vi "get DC test parameters.vi"(8 "error in (no error)":errorcluster, 10 "Step":T2=1 min=1 max=99 step=1, 11 "VISA Refnum in":refnum<visa-resource-name>) -> (0 "error out":errorcluster, 3 "VISA Refnum out":refnum<visa-resource-name>, 5 "DC Parameters":T1 {"Voltage Level [V]" min=50 max=6000 step=1 format="%.3p"; "Hi Limit [A]" min=1e-07 max=0.01 step=1e-07 format="%.2p"; "Test Time [s]" min=0.0 max=999.0 step=0.1 format="%.1p"; "Dwell Time [s]" min=0.0 max=999.0 step=0.1 format="%.1p"; "Lo Limit [A]" min=0.0 max=0.01 step=1e-06 format="%.2p"; "ARC Limit [A]" min=0.0 max=0.01 step=0.001 format="%.1p"; "Ramp Time [s]" min=0.0 max=999.0 step=0.1 format="%.1p"; "Fall Time [s]" min=0.0 max=999.0 step=0.1 format="%.1p"})   [LabVIEW 2025]
uses:
  <instrlib>/Chroma 19052/Public/Utility/Type Def/steps--numeric.ctl
  DC parameters--cluster.ctl
  <instrlib>/Chroma 19052/Public/Utility/Type Def/AC-DC-IR modes--ring.ctl
  <instrlib>/Chroma 19052/Public/Utility/Type Def/AC-DC modes--ring.ctl
  <instrlib>/Chroma 19052/Public/Utility/Type Def/DC-IR modes--ring.ctl
  <instrlib>/Chroma 19052/Chroma 19052.lvlib
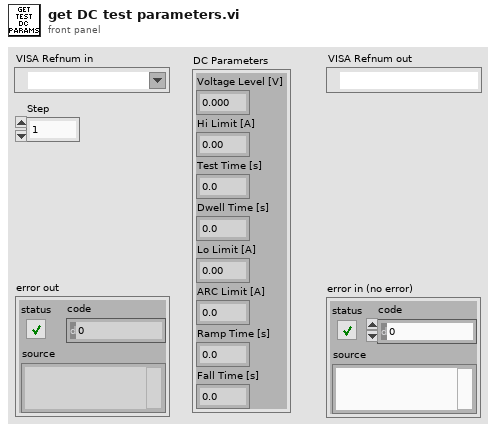
[diagram p1: front panel]
types:
  T1 = typedef "DC parameters--cluster.ctl" = cluster{"Voltage Level [V]":u16, "Hi Limit [A]":dbl, "Test Time [s] ":dbl, "Dwell Time [s]":dbl, "Lo Limit [A]":dbl, "ARC Limit [A]":dbl, "Ramp Time [s] ":dbl, "Fall Time [s]":dbl}
  T2 = typedef "Chroma 19052.lvlib/steps--numeric.ctl" = u8
  T3 = typedef "DC-IR modes--ring.ctl" = u16
  T4 = typedef "AC-DC modes--ring.ctl" = i32
  T5 = typedef "AC-DC-IR modes--ring.ctl" = u16
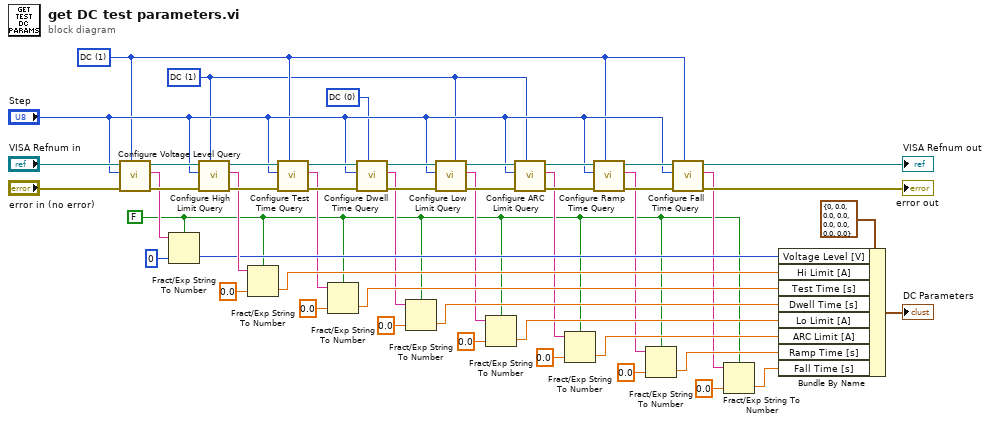
[diagram p0: block diagram]
diagram:
  w1 = FALSE
  w30 = T3 0 items=["DC", "IR"] ("Mode")
  w28 = T4 1 items=["AC", "DC"] ("Mode")
  w29 = T5 1 items=["AC", "DC", "IR"] ("Mode")
  n1 = call <instrlib>:"Configure Voltage Level Query.vi"("Mode"=w29, "error in (no error)"="error in (no error)", "Step"="Step", "VISA resource name"="VISA Refnum in") -> ("error out"=w38:errorcluster, "Voltage value [V]"=w25:string, "VISA resource name out"=w35:refnum<visa-resource-name>)  [unwired: 5 in]
  n2 = Fract/Exp String To Number(use system decimal point (T)=w1, string=w25, default (0 dbl)=u16 0 ("Voltage Level [V]")) -> (number=w21:u16)  [unwired: 1 in, 1 out]
  n3 = call <instrlib>:"Configure High Limit Query.vi"("Mode"=w28, "error in (no error)"=w38, "Step"="Step", "VISA resource name"=w35) -> ("error out"=w45:errorcluster, "High value [A]"=w22:string, "VISA resource name out"=w46:refnum<visa-resource-name>)  [unwired: 5 in]
  n4 = Fract/Exp String To Number(use system decimal point (T)=w1, string=w22, default (0 dbl)=0.0 ("Voltage Level [V]")) -> (number=w20:dbl)  [unwired: 1 in, 1 out]
  n5 = call <instrlib>:"Configure Test Time Query.vi"("Mode"=w29, "error in (no error)"=w45, "Step"="Step", "VISA resource name"=w46) -> ("error out"=w48:errorcluster, "Test Time value [s]"=w13:string, "VISA resource name out"=w32:refnum<visa-resource-name>)  [unwired: 5 in]
  n6 = Fract/Exp String To Number(use system decimal point (T)=w1, string=w13, default (0 dbl)=0.0 ("Voltage Level [V]")) -> (number=w12:dbl)  [unwired: 1 in, 1 out]
  n7 = call <instrlib>:"Configure Dwell Time Query.vi"("Mode"=w30, "error in (no error)"=w48, "Step"="Step", "VISA resource name"=w32) -> ("error out"=w47:errorcluster, "Dwell time value [s]"=w11:string, "VISA resource name out"=w49:refnum<visa-resource-name>)  [unwired: 5 in]
  n8 = Fract/Exp String To Number(use system decimal point (T)=w1, string=w11, default (0 dbl)=0.0 ("Voltage Level [V]")) -> (number=w10:dbl)  [unwired: 1 in, 1 out]
  n9 = call <instrlib>:"Configure Low Limit Query.vi"("Mode"=w28, "error in (no error)"=w47, "Step"="Step", "VISA resource name"=w49) -> ("error out"=w39:errorcluster, "Low value [A]"=w9:string, "VISA resource name out"=w40:refnum<visa-resource-name>)  [unwired: 5 in]
  n10 = Fract/Exp String To Number(use system decimal point (T)=w1, string=w9, default (0 dbl)=0.0 ("Voltage Level [V]")) -> (number=w8:dbl)  [unwired: 1 in, 1 out]
  n11 = call <instrlib>:"Configure ARC Limit Query.vi"("Mode"=w28, "error in (no error)"=w39, "Step"="Step", "VISA resource name"=w40) -> ("error out"=w41:errorcluster, "ARC Limit value [A]"=w7:string, "VISA resource name out"=w43:refnum<visa-resource-name>)  [unwired: 5 in]
  n12 = Fract/Exp String To Number(use system decimal point (T)=w1, string=w7, default (0 dbl)=0.0 ("Voltage Level [V]")) -> (number=w6:dbl)  [unwired: 1 in, 1 out]
  n13 = call <instrlib>:"Configure Ramp Time Query.vi"("Mode"=w29, "error in (no error)"=w41, "Step"="Step", "VISA resource name"=w43) -> ("error out"=w42:errorcluster, "Ramp Time value [s]"=w5:string, "VISA resource name out"=w44:refnum<visa-resource-name>)  [unwired: 5 in]
  n14 = Fract/Exp String To Number(use system decimal point (T)=w1, string=w5, default (0 dbl)=0.0 ("Voltage Level [V]")) -> (number=w4:dbl)  [unwired: 1 in, 1 out]
  n15 = call <instrlib>:"Configure Fall Time Query.vi"("Mode"=w29, "error in (no error)"=w42, "Step"="Step", "VISA resource name"=w44) -> ("error out"=→"error out":errorcluster, "Fall Time value"=w3:string, "VISA resource name out"=→"VISA Refnum out":refnum<visa-resource-name>)  [unwired: 5 in]
  n16 = Fract/Exp String To Number(use system decimal point (T)=w1, string=w3, default (0 dbl)=0.0 ("Voltage Level [V]")) -> (number=w2:dbl)  [unwired: 1 in, 1 out]
  n17 = Bundle By Name(cluster=T1 {"Voltage Level [V]"=0, "Hi Limit [A]"=0.0, "Test Time [s] "=0.0, "Dwell Time [s]"=0.0, "Lo Limit [A]"=0.0, "ARC Limit [A]"=0.0, "Ramp Time [s] "=0.0, "Fall Time [s]"=0.0} ("DC Parameters"), "Voltage Level [V]"=w21, "Hi Limit [A]"=w20, "Test Time [s]"=w12, "Dwell Time [s]"=w10, "Lo Limit [A]"=w8, "ARC Limit [A]"=w6, "Ramp Time [s]"=w4, "Fall Time [s]"=w2) -> (→"DC Parameters":T1)
